vi "Form_设备通讯配置 Start Module.vi"(8 "error in (no error)":errorcluster caption="错误输入（无错误）") -> (0 "error out":errorcluster caption="错误输出", 3 "VI引用句柄":refnum<vi>)   [LabVIEW 2018]
uses:
  Basic Library/Module Admin_class/lib_QMH_Module_Admin.lvclass
  Basic Library/Module Admin_class/lib_QMH_Module_Admin.lvclass/lib_QMH_Module_Admin.ctl
  Basic Library/Module Admin_class/lib_QMH_Set External Launch.vi
  <vilib>/Utility/error.llb/Error Cluster From Error Code.vi
  <vilib>/ErrorRing/Error Ring.xnode
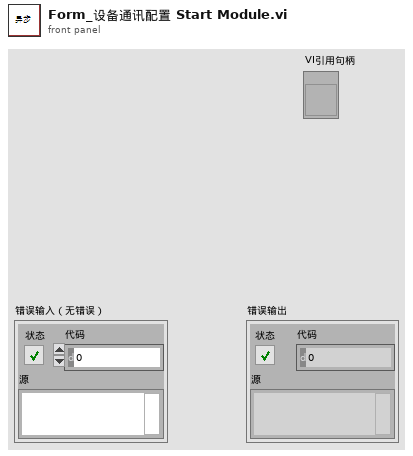
[diagram p1: front panel]
types:
  T1 = enum32{"Bad", "Idle", "Run top level", "Running"}
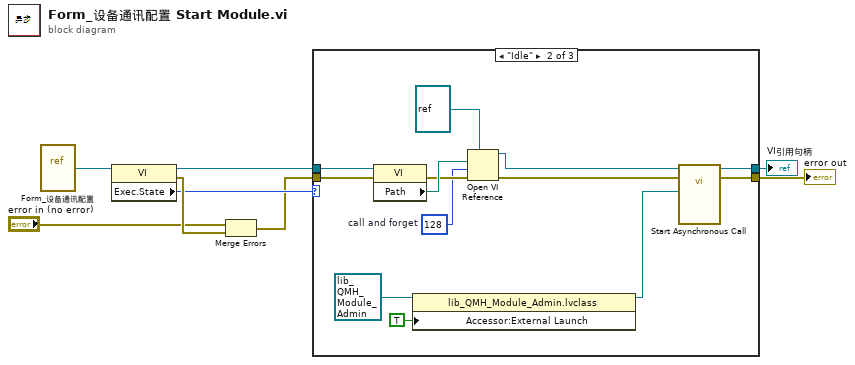
[diagram p0: block diagram]
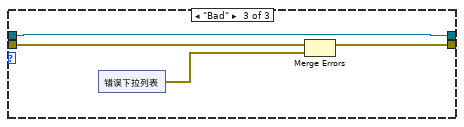
[diagram p3: hidden frame]
diagram:
  n1 = vi-ref "Form_设备通讯配置.vi"() -> (w1:refnum<vi>)
  n2 = property class="VI"(reference=w1) -> (reference out=w6:refnum<vi>, error out=w8:errorcluster, "Exec.State"=w7:T1)  [unwired: 1 in]
  n3 = Merge Errors("error in (no error)", w8) -> (w5:errorcluster)
  n4 = case shown="\"Idle\"" w7 {
    tunnel: w6 -> [w9 w21 w24]
    tunnel: w5 -> [w10 w20 w25]
    tunnel: [w10 w14 w26] -> w4
    tunnel: [w9 w15 w24] -> w3
    frame "Run top level", "Running" {
    }
    frame "Idle" {
      w19 = 128  # call and forget
      n5 = property class="VI"(reference=w21, error in=w20) -> (error out=w22:errorcluster, "Path"=w23:path)  [unwired: 1 out]
      n6 = property class="lib_QMH_Module_Admin.lvclass"(reference=refnum<class "lib_QMH_Module_Admin.lvclass"> refnum ("Module Admin"), "Accessor:External Launch"=TRUE ("External Launch")) -> (reference out=w11:refnum<class "lib_QMH_Module_Admin.lvclass">)  [unwired: 1 in, 1 out]
      n7 = Open VI Reference(type specifier VI Refnum (for type only)=refnum<vi> refnum, vi path=w23, options=w19, error in (no error)=w22) -> (vi reference=w16:refnum<vi>, error out=w17:errorcluster)  [unwired: 2 in]
      n8 = call-by-ref "Start Asynchronous Call"(reference=w16, error in=w17, "Module Admin"=w11) -> (reference out=w15:refnum<vi>, error out=w14:errorcluster)  [unwired: 11 in]
    }
    frame "Bad" {
      n9 = xnode "错误下拉列表"() -> ("错误输出"=w27:errorcluster)
      n10 = Merge Errors(w25, w27) -> (w26:errorcluster)
    }
  }
  "error out" <- w4
  "VI引用句柄" <- w3
